vi "ReadMemory.vi"(2 "Address":i32, 3 "Board":T1(ring)=enum."TIMING_BOARD", 4 "Type":enum16{"X", "Y", "P", "R", "D"}(ring)) -> (0 "Value":i32, 1 "Error":bool)   [LabVIEW 2014]
panel:
  out "Hex Address":i32 format="%.0x"
  out "Hex Value":i32 format="%.0x"
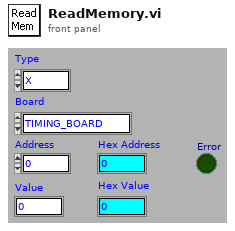
[diagram p1: front panel]
types:
  T1 = enum32{"not used", "PCI_BOARD", "TIMING_BOARD", "UTILITY_BOARD"}
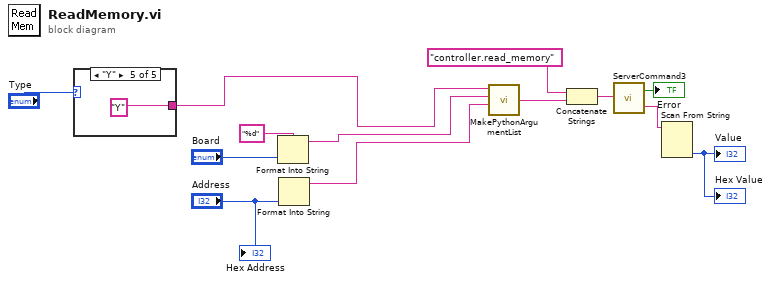
[diagram p0: block diagram]
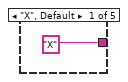
[diagram p2: hidden frame]
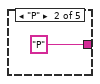
[diagram p3: hidden frame]
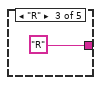
[diagram p4: hidden frame]
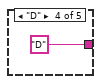
[diagram p5: hidden frame]
diagram:
  n1 = case shown="\"Y\"" "Type" {
    tunnel: ["X" "P" "R" "D" "Y"] -> w1
    frame "X", Default {
    }
    frame "P" {
    }
    frame "R" {
    }
    frame "D" {
    }
    frame "Y" {
    }
  }
  n2 = Format Into String(format string="%d" ("Format String"), "Board") -> (resulting string=w7:string)  [unwired: 2 in, 1 out]
  n3 = Format Into String("Address") -> (resulting string=w6:string)  [unwired: 3 in, 1 out]
  n4 = call "MakePythonArgumentList.vi"("Arg 3"=w6, "Arg 2"=w7, "Arg 1"=w1) -> ("Args Out"=w4:string)  [unwired: 3 in]
  n5 = Concatenate Strings("controller.read_memory" ("string"), w4) -> (w3:string)
  n6 = call "ServerCommand3.vi"("Command"=w3) -> ("Error"=→"Error":bool, "Reply"=w2:string)
  n7 = Scan From String(input string=w2) -> (output 1=→"Value" →"Hex Value":i32)  [unwired: 4 in, 3 out]
  "Hex Address" <- "Address"
